vi "Periodic Tasks.vi"(8 "error in":errorcluster) -> ()   [LabVIEW 2014]
doc: "This VI runs in parallel to other tasks. It can contain as many user-defined periodic loops as you need. These can carry out PID or other sorts of timed response."
uses:
  <vilib>/Rock Robotics/WPI/Joystick/WPI_JoystickGetSetRefNum.vi
  <vilib>/Rock Robotics/WPI/RobotDrive/WPI_RobotDriveGetSetRefNum.vi
  Global Variables.vi
  <vilib>/addons/control/pid/NI_PID_pid.lvlib
  <vilib>/addons/control/pid/pid.llb/PID (DBL).vi
panel:
  in  "constant":dbl
  out "encoder counts per iteration 2":dbl format="%#_12g"
  in  "motor speed 2":dbl
  in  "total iterations 2":dbl
  out "iterations":dbl
  out "encoder counts per iteration":dbl format="%#_12g"
  in  "motor speed":dbl
  in  "total iterations":dbl
  out "encoder count left":dbl
  out "encoder count right":dbl
  out "left to target difference":dbl
  out "Waveform Graph 2":dbl[](graph)
  in  "reset graph":bool
  out "Waveform Graph":dbl[](graph)
  in  "move to distance":dbl
  in  "right PID gains":T1={"proportional gain (Kc)"=1.0, "integral time (Ti, min)"=0.01, "derivative time (Td, min)"=0.0} {"derivative time (Td, min)" format="%.4f"; "integral time (Ti, min)" format="%.6f"; "proportional gain (Kc)" format="%.5f"}
  in  "left PID gains":T1={"proportional gain (Kc)"=1.0, "integral time (Ti, min)"=0.01, "derivative time (Td, min)"=0.0} {"derivative time (Td, min)" format="%.10f"; "integral time (Ti, min)" format="%.3f"; "proportional gain (Kc)" format="%.5f"}
  in  "right output range":cluster{"output high":dbl, "output low":dbl}={"output high"=100.0, "output low"=-100.0} {"output low" format="%.2f"; "output high" format="%.2f"}
  in  "left output range":cluster{"output high":dbl, "output low":dbl}={"output high"=100.0, "output low"=-100.0} {"output low" format="%.2f"; "output high" format="%.2f"}
  out "Maximum Difference":dbl
  in  "Distance PID":T1={"proportional gain (Kc)"=1.0, "integral time (Ti, min)"=0.01, "derivative time (Td, min)"=0.0} {"derivative time (Td, min)" format="%.3f"; "integral time (Ti, min)" format="%.3f"; "proportional gain (Kc)" format="%.3f"}
  in  "Difference PID":T1={"proportional gain (Kc)"=1.0, "integral time (Ti, min)"=0.01, "derivative time (Td, min)"=0.0} {"derivative time (Td, min)" format="%.3f"; "integral time (Ti, min)" format="%.3f"; "proportional gain (Kc)" format="%.3f"}
  out "Right Encoder Value":dbl
  out "Left Encoder Value":dbl
  in  "PID gains":T1={"proportional gain (Kc)"=1.0, "integral time (Ti, min)"=0.01, "derivative time (Td, min)"=0.0} {"derivative time (Td, min)" format="%.3f"; "integral time (Ti, min)" format="%.3f"; "proportional gain (Kc)" format="%.3f"}
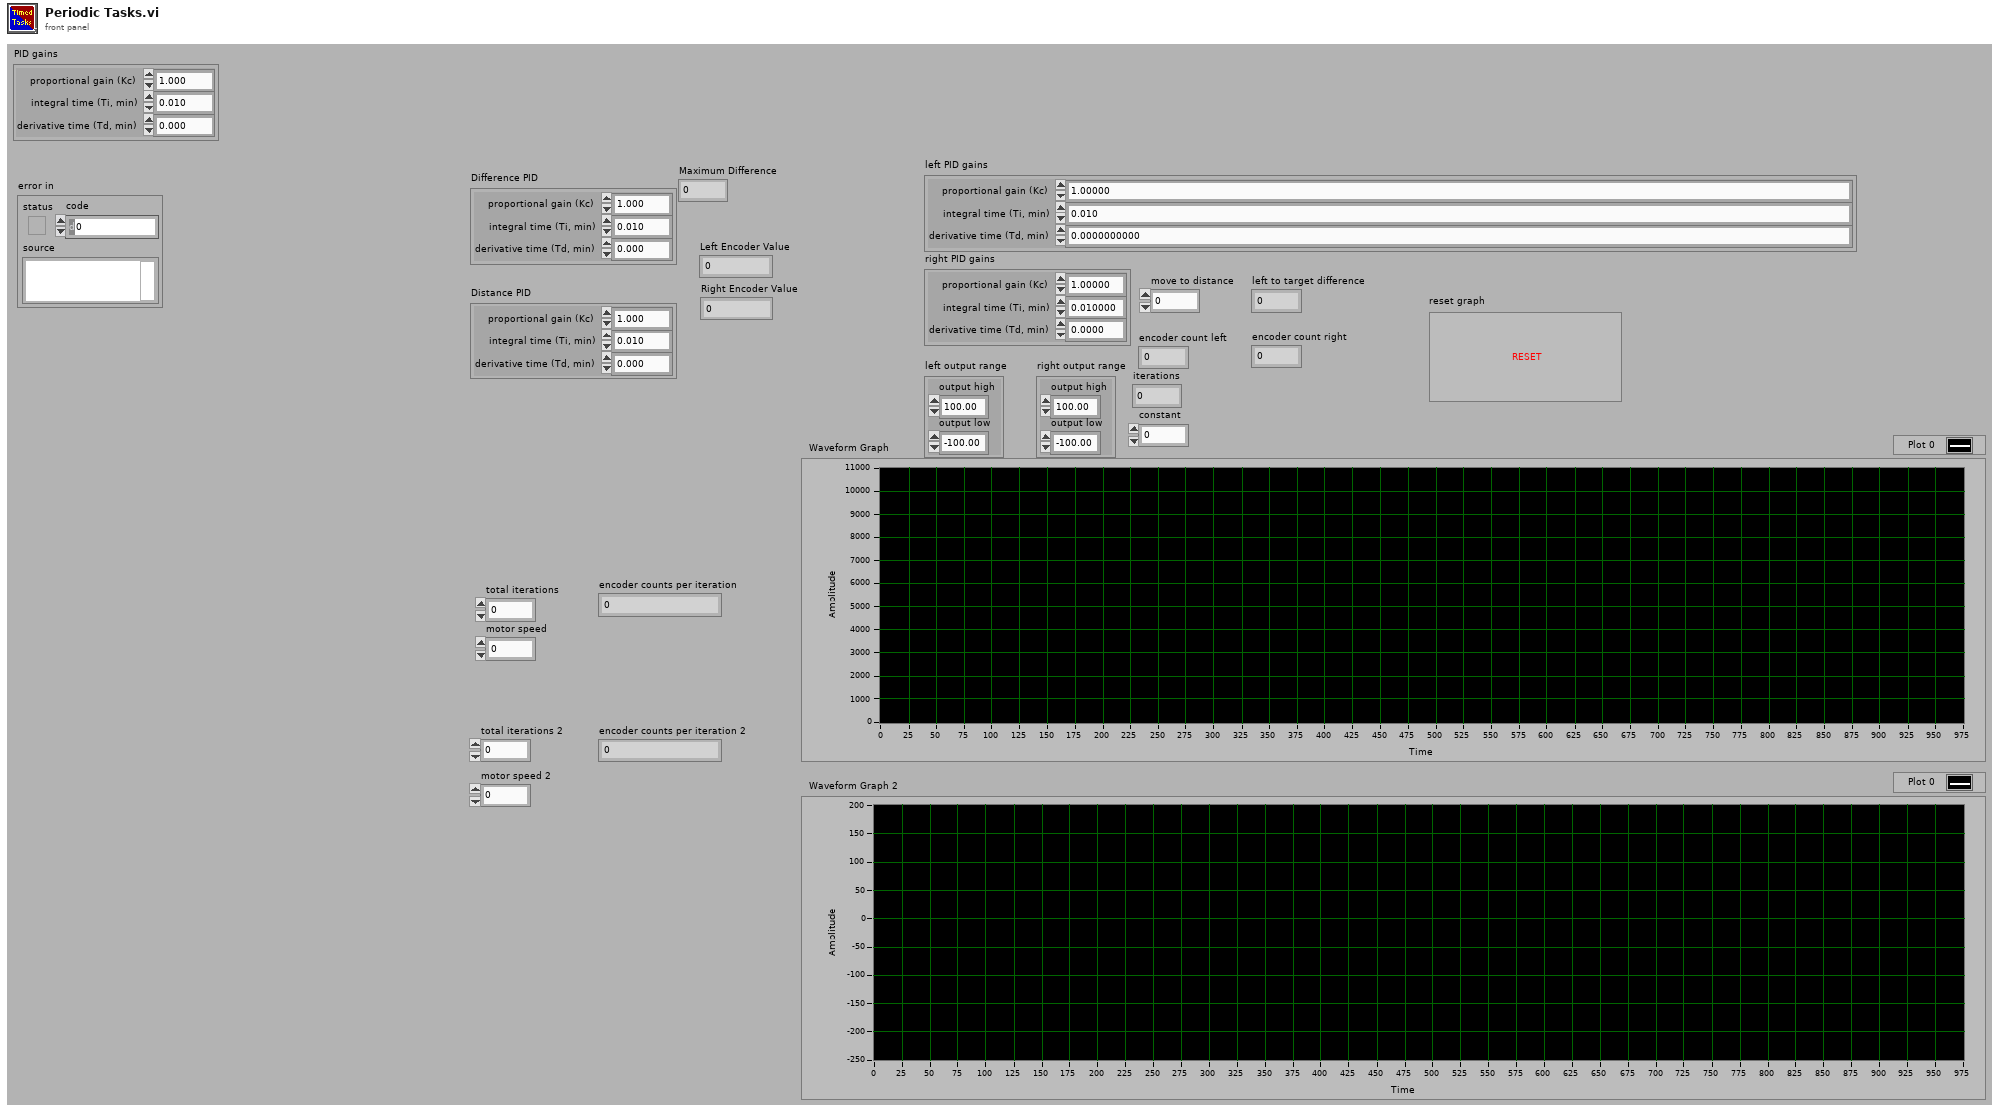
[diagram p1: front panel]
types:
  T1 = cluster{"proportional gain (Kc)":dbl, "integral time (Ti, min)":dbl, "derivative time (Td, min)":dbl}
  T2 = typedef "WPI_JoystickDevRef.ctl" = cluster{"Device":T3}
  T3 = typedef "WPI_JoystickDeviceEnum.ctl" = enum16{"USB 0", "USB 1", "USB 2", "USB 3", "USB 4", "USB 5"}
  T4 = typedef "WPI_RobotDriveDevRef.ctl" = cluster{"DevStatus":errorcluster, "Motors[]":T5[], "Square Inputs":bool, "Max Output":dbl}
  T5 = typedef "WPI_MotorControlDeviceRef.ctl" = cluster{"DeviceStatus":errorcluster, "Type":T6, "PWM":cluster{"Controller":T7, "PWM Channel":T8, "DeadBand":T9}, "CAN":cluster{"Device Number":u8, "Control Mode":T10, "Semaphore":T11, "Max Vout":dbl, "TalonSRX Control Mode":T12}, "Invert":bool, "TransformRef":T13, "InvTransformRef":T13}
  T6 = typedef "WPI_MotorControlType.ctl" = enum16{"PWM", "CAN", "CANTalonSRX"}
  T7 = typedef "FPGA_TypedefDigitalModule.ctl" = enum16{"Controller 1"}
  T8 = typedef "FPGA_DIOPWMChannel.ctl" = enum8{"PWM 0", "PWM 1", "PWM 2", "PWM 3", "PWM 4", "PWM 5", "PWM 6", "PWM 7", "PWM 8", "PWM 9", "PWM MXP 0", "PWM MXP 1", "PWM MXP 2", "PWM MXP 3", "PWM MXP 4", "PWM MXP 5", "PWM MXP 6", "PWM MXP 7", "PWM MXP 8", "PWM MXP 9", "Invalid"}
  T9 = typedef "WPI_PWMDeadband.ctl" = cluster{"Name":string, "maxPositivePwm":i32, "minPositivePwm":i32, "centerPwm":i32, "maxNegativePwm":i32, "minNegativePwm":i32, "angularRange":u16}
  T10 = typedef "WPI_CANJaguar_ControlMode.ctl" = enum8{"Percent VBus", "Current", "Speed", "Position", "Voltage"}
  T11 = typedef "Semaphore RefNum" = refnum<k1>
  T12 = typedef "WPI_CANTalonSRX_APIControlMode.ctl" = enum8{"Percent VBus", "Speed", "Position", "Slave", "Unchanged / Invalid"}
  T13 = typedef "WPI_PWMTransform_ConPane.ctl" = refnum<vi>
  T14 = cluster{"JoystickDevRef":T2, "RobotDriveDevRef":T4}
  T15 = typedef "WPI_EncoderDevRef.ctl" = cluster{"DevStatus":errorcluster, "EncoderIndex":T16, "CounterIndex":T17, "DistancePerCount":dbl, "Decoding Type":T18}
  T16 = typedef "FPGA_EncoderIdx.ctl" = enum8{"Enc 0", "Enc 1", "Enc 2", "Enc 3", "Enc 4", "Enc 5", "Enc 6", "Enc 7", "Invalid"}
  T17 = typedef "FPGA_CounterCtrSystemIndex.ctl" = enum8{"Ctr 0", "Ctr 1", "Ctr 2", "Ctr 3", "Ctr 4", "Ctr 5", "Ctr 6", "Ctr 7", "Invalid"}
  T18 = typedef "WPI_EncoderType.ctl" = enum16{"1x", "2x", "4x"}
  T19 = enum16{"Stop", "Three Tote", "Two Tote", "One Tote", "Step", "Top", "Home", "Joystick", "Joystick Slave", "D Pad"}
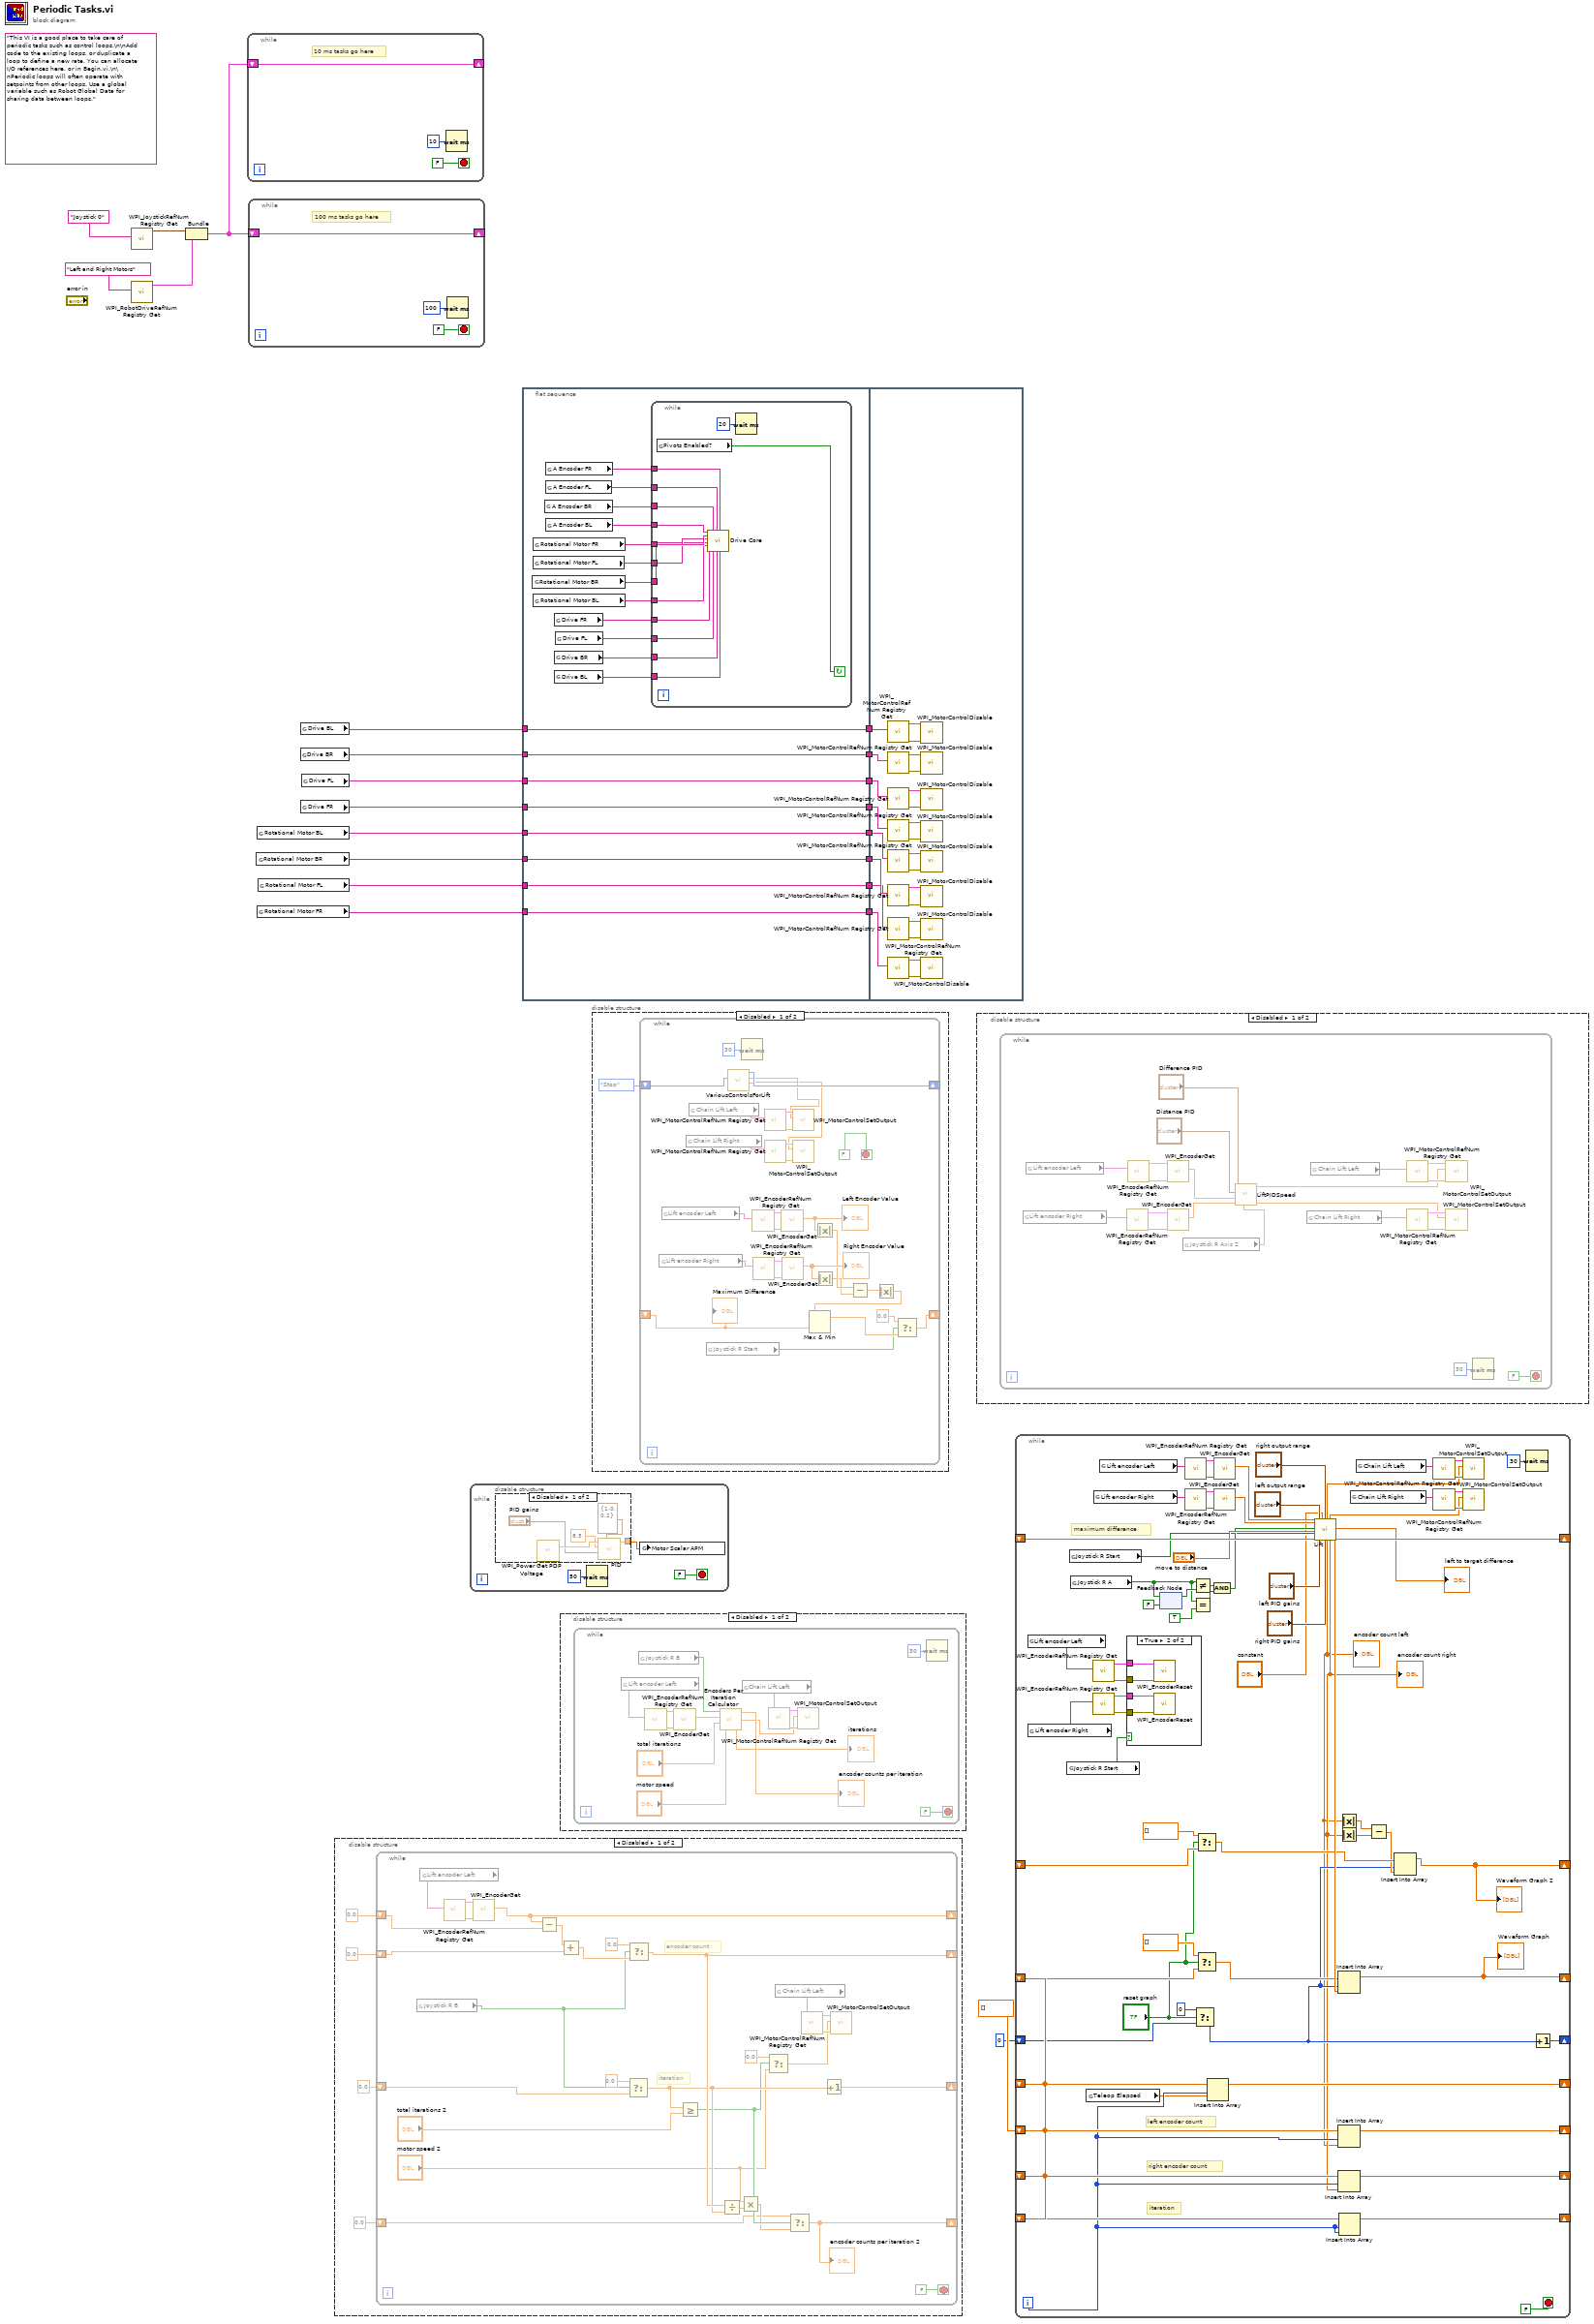
[diagram p0: block diagram]
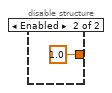
[diagram p7: hidden frame]
diagram:
  w2 = dbl[] []
  (unwired) "This VI is a good place to take care of periodic tasks such as control loops.\n\nAdd code to the existing loops, or duplicate a loop to define a new rate. You can allocate I/O references here, or in Begin.vi.\n\nPeriodic loops will often operate with setpoints from other loops. Use a global variable such as Robot Global Data for sharing data between loops."
  n1 = call <vilib>:"WPI_JoystickRefNum Registry Get.vi"("refnum name"="Joystick 0") -> ("JoystickDevRef"=w21:T2)  [unwired: 1 in, 9 out]
  n2 = call <vilib>:"WPI_RobotDriveRefNum Registry Get.vi"("refnum name"="Left and Right Motors") -> ("RobotDriveDevRef"=w20:T4)  [unwired: 1 in, 9 out]
  n3 = Bundle("JoystickDevRef"=w21, "RobotDriveDevRef"=w20) -> (w19:T14)  [unwired: 1 out]
  n4 = while {
    shift-right: [w24] -> _
    shift-left: w19 -> [w24]
    stop <- FALSE stop-if-true
    # "10 ms tasks go here"
    n5 = Wait (ms)(milliseconds to wait=u32 10) -> ()  [unwired: 1 out]
  }
  n6 = while {
    shift-right: [w27] -> _
    shift-left: w19 -> [w27]
    stop <- FALSE stop-if-true
    # "100 ms tasks go here"
    n7 = Wait (ms)(milliseconds to wait=u32 100) -> ()  [unwired: 1 out]
  }
  n8 = global read "Global Variables.vi" "Rotational Motor BR"() -> (w7:string)
  n9 = global read "Global Variables.vi" "Rotational Motor BL"() -> (w9:string)
  n10 = global read "Global Variables.vi" "Rotational Motor FR"() -> (w3:string)
  n11 = global read "Global Variables.vi" "Rotational Motor FL"() -> (w5:string)
  n12 = global read "Global Variables.vi" "Drive BR"() -> (w15:string)
  n13 = global read "Global Variables.vi" "Drive BL"() -> (w17:string)
  n14 = global read "Global Variables.vi" "Drive FR"() -> (w11:string)
  n15 = global read "Global Variables.vi" "Drive FL"() -> (w13:string)
  n16 = disable-structure shown="Disabled" {
    frame Disabled {
      n17 = while {
        shift-right: [w60] -> _
        shift-left: 0.0 -> [w59]
        shift-right: [w45] -> _
        shift-left: 0.0 -> [w46]
        shift-right: [w50] -> _
        shift-left: 0.0 -> [w51]
        shift-right: [w36] -> _
        shift-left: 0.0 -> [w37]
        stop <- FALSE stop-if-true
        # "iteration"
        # "encoder count"
        n18 = global read "Global Variables.vi" "Joystick R B"() -> (w34:bool)
        n19 = global read "Global Variables.vi" "Lift encoder Left"() -> (w55:string)
        n20 = call <vilib>:"WPI_EncoderRefNum Registry Get.vi"("refnum name"=w55) -> ("error out"=w56:errorcluster, "EncoderDevRef"=w57:T15)  [unwired: 9 in]
        n21 = call <vilib>:"WPI_EncoderGet.vi"("error in (no error)"=w56, "EncoderDevRef"=w57) -> ("Distance"=w50:dbl)  [unwired: 4 in, 5 out]
        n22 = Subtract(x=w50, y=w51) -> (x-y=w49:dbl)
        n23 = Add(x=w49, y=w46) -> (x+y=w48:dbl)
        n24 = Select(t=0.0, s=w34, f=w59) -> (s? t:f=w44:dbl)
        n25 = Select(t=0.0, s=w34, f=w48) -> (s? t:f=w45:dbl)
        n26 = Greater Or Equal?(x=w44, y="total iterations 2") -> (x >= y?=w41:bool)
        n27 = Divide(x=w45, y=w44) -> (x/y=w40:dbl)
        n28 = Multiply(x="motor speed 2", y=w40) -> (x*y=w38:dbl)
        n29 = Select(t=0.0, s=w41, f="motor speed 2") -> (s? t:f=w35:dbl)
        n30 = global read "Global Variables.vi" "Chain Lift Left"() -> (w54:string)
        n31 = Select(t=w37, s=w41, f=w38) -> (s? t:f=w36:dbl)
        "encoder counts per iteration 2" <- w36
        n32 = call <vilib>:"WPI_MotorControlRefNum Registry Get.vi"("refnum name"=w54) -> ("error out"=w52:errorcluster, "MotorControlDevRef"=w53:T5)  [unwired: 9 in]
        n33 = Increment(x=w44) -> (x+1=w60:dbl)
        n34 = call <vilib>:"WPI_MotorControlSetOutput.vi"("error in (no error)"=w52, "Output"=w35, "MotorControlDevRef"=w53) -> ()  [unwired: 6 in, 3 out]
      }
    }
    frame Enabled {
    }
  }
  n35 = while {
    stop <- FALSE stop-if-true
    n36 = disable-structure shown="Disabled" {
      disable-tunnel: [w65 1.0 ("Motor Scalar APM")] -> w62
      frame Disabled {
        n37 = call <vilib>:"WPI_Power Get PDP Voltage.vi"() -> ("voltage (V)"=w68:dbl)  [unwired: 14 in, 1 out]
        n38 = call-poly <vilib>:"PID.vi"("output range"=cluster{"output high":dbl, "output low":dbl} {"output high"=1.0, "output low"=0.2}, "PID gains"="PID gains", "process variable"=8.5 ("setpoint"), "setpoint"=w68) -> ("output"=w65:dbl)  [unwired: 6 in, 1 out]
      }
      frame Enabled {
      }
    }
    n39 = Wait (ms)(milliseconds to wait=u32 50) -> ()  [unwired: 1 out]
    n40 = global write "Global Variables.vi" "Motor Scalar APM"(w62) -> ()
  }
  n41 = flat-sequence {
    tunnel: [w78] -> w18
    tunnel: w17 -> [w78]
    tunnel: [w77] -> w16
    tunnel: w15 -> [w77]
    tunnel: [w76] -> w14
    tunnel: w13 -> [w76]
    tunnel: [w75] -> w12
    tunnel: w11 -> [w75]
    tunnel: [w74] -> w10
    tunnel: w9 -> [w74]
    tunnel: [w73] -> w8
    tunnel: w7 -> [w73]
    tunnel: [w72] -> w6
    tunnel: w5 -> [w72]
    tunnel: [w71] -> w4
    tunnel: w3 -> [w71]
    tunnel: w18 -> [w112]
    tunnel: w16 -> [w111]
    tunnel: w14 -> [w110]
    tunnel: w12 -> [w109]
    tunnel: w10 -> [w108]
    tunnel: w8 -> [w107]
    tunnel: w6 -> [w106]
    tunnel: w4 -> [w105]
    frame #0 {
      n42 = global read "Global Variables.vi" "Rotational Motor BR"() -> (w84:string)
      n43 = global read "Global Variables.vi" "Rotational Motor FR"() -> (w86:string)
      n44 = global read "Global Variables.vi" "Rotational Motor FL"() -> (w85:string)
      n45 = global read "Global Variables.vi" "Rotational Motor BL"() -> (w83:string)
      n46 = global read "Global Variables.vi" "A Encoder BR"() -> (w88:string)
      n47 = global read "Global Variables.vi" "A Encoder FR"() -> (w90:string)
      n48 = global read "Global Variables.vi" "A Encoder FL"() -> (w89:string)
      n49 = global read "Global Variables.vi" "A Encoder BL"() -> (w87:string)
      n50 = global read "Global Variables.vi" "Drive FR"() -> (w82:string)
      n51 = global read "Global Variables.vi" "Drive BR"() -> (w80:string)
      n52 = global read "Global Variables.vi" "Drive BL"() -> (w79:string)
      n53 = global read "Global Variables.vi" "Drive FL"() -> (w81:string)
      n54 = while {
        tunnel: w90 -> [w103]
        tunnel: w89 -> [w102]
        tunnel: w88 -> [w101]
        tunnel: w87 -> [w100]
        tunnel: w86 -> [w99]
        tunnel: w85 -> [w98]
        tunnel: w84 -> [w97]
        tunnel: w83 -> [w96]
        tunnel: w82 -> [w95]
        tunnel: w81 -> [w94]
        tunnel: w80 -> [w93]
        tunnel: w79 -> [w92]
        stop <- w104 continue-if-true
        n55 = global read "Global Variables.vi" "Pivots Enabled?"() -> (w104:bool)
        n56 = call "Drive Core.vi"("A Encoder BL"=w100, "Rotational Motor FR"=w99, "Rotational Motor FL"=w98, "Rotational Motor BR"=w97, "Rotational Motor BL"=w96, "Drive Motor FR"=w95, "A Encoder BR"=w101, "Drive Motor FL"=w94, "A Encoder FL"=w102, "Drive Motor BR"=w93, "A Encoder FR"=w103, "Drive Motor BL"=w92) -> ()  [unwired: 8 in]
        n57 = Wait (ms)(milliseconds to wait=u32 20) -> ()  [unwired: 1 out]
      }
    }
    frame #1 {
      n58 = call <vilib>:"WPI_MotorControlRefNum Registry Get.vi"("refnum name"=w112) -> ("error out"=w128:errorcluster, "MotorControlDevRef"=w127:T5)  [unwired: 9 in]
      n59 = call <vilib>:"WPI_MotorControlRefNum Registry Get.vi"("refnum name"=w111) -> ("error out"=w126:errorcluster, "MotorControlDevRef"=w125:T5)  [unwired: 9 in]
      n60 = call <vilib>:"WPI_MotorControlRefNum Registry Get.vi"("refnum name"=w110) -> ("error out"=w124:errorcluster, "MotorControlDevRef"=w123:T5)  [unwired: 9 in]
      n61 = call <vilib>:"WPI_MotorControlRefNum Registry Get.vi"("refnum name"=w109) -> ("error out"=w122:errorcluster, "MotorControlDevRef"=w121:T5)  [unwired: 9 in]
      n62 = call <vilib>:"WPI_MotorControlRefNum Registry Get.vi"("refnum name"=w108) -> ("error out"=w120:errorcluster, "MotorControlDevRef"=w119:T5)  [unwired: 9 in]
      n63 = call <vilib>:"WPI_MotorControlRefNum Registry Get.vi"("refnum name"=w107) -> ("error out"=w118:errorcluster, "MotorControlDevRef"=w117:T5)  [unwired: 9 in]
      n64 = call <vilib>:"WPI_MotorControlRefNum Registry Get.vi"("refnum name"=w106) -> ("error out"=w116:errorcluster, "MotorControlDevRef"=w115:T5)  [unwired: 9 in]
      n65 = call <vilib>:"WPI_MotorControlRefNum Registry Get.vi"("refnum name"=w105) -> ("error out"=w114:errorcluster, "MotorControlDevRef"=w113:T5)  [unwired: 9 in]
      n66 = call <vilib>:"WPI_MotorControlDisable.vi"("error in (no error)"=w128, "MotorControlDevRef"=w127) -> ()  [unwired: 8 in, 2 out]
      n67 = call <vilib>:"WPI_MotorControlDisable.vi"("error in (no error)"=w126, "MotorControlDevRef"=w125) -> ()  [unwired: 8 in, 2 out]
      n68 = call <vilib>:"WPI_MotorControlDisable.vi"("error in (no error)"=w124, "MotorControlDevRef"=w123) -> ()  [unwired: 8 in, 2 out]
      n69 = call <vilib>:"WPI_MotorControlDisable.vi"("error in (no error)"=w122, "MotorControlDevRef"=w121) -> ()  [unwired: 8 in, 2 out]
      n70 = call <vilib>:"WPI_MotorControlDisable.vi"("error in (no error)"=w120, "MotorControlDevRef"=w119) -> ()  [unwired: 8 in, 2 out]
      n71 = call <vilib>:"WPI_MotorControlDisable.vi"("error in (no error)"=w118, "MotorControlDevRef"=w117) -> ()  [unwired: 8 in, 2 out]
      n72 = call <vilib>:"WPI_MotorControlDisable.vi"("error in (no error)"=w116, "MotorControlDevRef"=w115) -> ()  [unwired: 8 in, 2 out]
      n73 = call <vilib>:"WPI_MotorControlDisable.vi"("error in (no error)"=w114, "MotorControlDevRef"=w113) -> ()  [unwired: 8 in, 2 out]
    }
  }
  n74 = disable-structure shown="Disabled" {
    frame Disabled {
      n75 = while {
        stop <- FALSE stop-if-true
        n76 = global read "Global Variables.vi" "Lift encoder Left"() -> (w143:string)
        n77 = global read "Global Variables.vi" "Joystick R B"() -> (w130:bool)
        n78 = call <vilib>:"WPI_EncoderRefNum Registry Get.vi"("refnum name"=w143) -> ("error out"=w142:errorcluster, "EncoderDevRef"=w141:T15)  [unwired: 9 in]
        n79 = call <vilib>:"WPI_EncoderGet.vi"("error in (no error)"=w142, "EncoderDevRef"=w141) -> ("Distance"=w137:dbl)  [unwired: 4 in, 5 out]
        n80 = call "Encoders Per Iteration Calculator.vi"("motor speed"="motor speed", "total iterations"="total iterations", "encoder count"=w137, "go"=w130) -> ("iterations"=→"iterations":dbl, "motor speed out"=w132:dbl, "encoder counts per iteration"=→"encoder counts per iteration":dbl)
        n81 = global read "Global Variables.vi" "Chain Lift Left"() -> (w138:string)
        n82 = call <vilib>:"WPI_MotorControlRefNum Registry Get.vi"("refnum name"=w138) -> ("error out"=w140:errorcluster, "MotorControlDevRef"=w139:T5)  [unwired: 9 in]
        n83 = call <vilib>:"WPI_MotorControlSetOutput.vi"("error in (no error)"=w140, "Output"=w132, "MotorControlDevRef"=w139) -> ()  [unwired: 6 in, 3 out]
        n84 = Wait (ms)(milliseconds to wait=u32 30) -> ()  [unwired: 1 out]
      }
    }
    frame Enabled {
    }
  }
  n85 = disable-structure shown="Disabled" {
    frame Disabled {
      n86 = while {
        shift-right: [w172] -> _
        shift-left: T19."Stop" ("State Out") -> [w162]
        shift-right: [w148] -> _
        shift-left: _ -> [w149]
        stop <- FALSE stop-if-true
        n87 = global read "Global Variables.vi" "Lift encoder Right"() -> (w156:string)
        n88 = global read "Global Variables.vi" "Lift encoder Left"() -> (w161:string)
        n89 = global read "Global Variables.vi" "Chain Lift Right"() -> (w166:string)
        n90 = global read "Global Variables.vi" "Chain Lift Left"() -> (w167:string)
        n91 = global read "Global Variables.vi" "Joystick R Start"() -> (w145:bool)
        n92 = call "VariousControlsForLift.vi"("State"=w162) -> ("Lift Motor Right"=w163:dbl, "Lift Motor Left"=w168:dbl, "State Out"=w172:T19)  [unwired: 8 in]
        n93 = Wait (ms)(milliseconds to wait=u32 30) -> ()  [unwired: 1 out]
        n94 = call <vilib>:"WPI_EncoderRefNum Registry Get.vi"("refnum name"=w161) -> ("error out"=w160:errorcluster, "EncoderDevRef"=w159:T15)  [unwired: 9 in]
        n95 = call <vilib>:"WPI_EncoderRefNum Registry Get.vi"("refnum name"=w156) -> ("error out"=w157:errorcluster, "EncoderDevRef"=w158:T15)  [unwired: 9 in]
        n96 = call <vilib>:"WPI_MotorControlRefNum Registry Get.vi"("refnum name"=w167) -> ("error out"=w171:errorcluster, "MotorControlDevRef"=w170:T5)  [unwired: 9 in]
        n97 = call <vilib>:"WPI_MotorControlRefNum Registry Get.vi"("refnum name"=w166) -> ("error out"=w164:errorcluster, "MotorControlDevRef"=w165:T5)  [unwired: 9 in]
        n98 = call <vilib>:"WPI_EncoderGet.vi"("error in (no error)"=w160, "EncoderDevRef"=w159) -> ("Distance"=w155:dbl)  [unwired: 4 in, 5 out]
        "Left Encoder Value" <- w155
        n99 = call <vilib>:"WPI_EncoderGet.vi"("error in (no error)"=w157, "EncoderDevRef"=w158) -> ("Distance"=w154:dbl)  [unwired: 4 in, 5 out]
        "Right Encoder Value" <- w154
        n100 = call <vilib>:"WPI_MotorControlSetOutput.vi"("error in (no error)"=w171, "Output"=w168, "MotorControlDevRef"=w170) -> ()  [unwired: 6 in, 3 out]
        n101 = call <vilib>:"WPI_MotorControlSetOutput.vi"("error in (no error)"=w164, "Output"=w163, "MotorControlDevRef"=w165) -> ()  [unwired: 6 in, 3 out]
        n102 = Absolute Value(x=w155) -> (abs(x)=w153:dbl)
        n103 = Absolute Value(x=w154) -> (abs(x)=w152:dbl)
        n104 = Subtract(x=w153, y=w152) -> (x-y=w151:dbl)
        n105 = Absolute Value(x=w151) -> (abs(x)=w150:dbl)
        n106 = Max & Min(x=w150, y=w149) -> (max(x,y)=w146:dbl)  [unwired: 1 out]
        n107 = Select(t=0.0 ("f"), s=w145, f=w146) -> (s? t:f=w148:dbl)
        "Maximum Difference" <- w149
      }
    }
    frame Enabled {
    }
  }
  n108 = disable-structure shown="Disabled" {
    frame Disabled {
      n109 = while {
        stop <- FALSE stop-if-true
        n110 = global read "Global Variables.vi" "Lift encoder Right"() -> (w185:string)
        n111 = global read "Global Variables.vi" "Lift encoder Left"() -> (w188:string)
        n112 = call <vilib>:"WPI_EncoderRefNum Registry Get.vi"("refnum name"=w185) -> ("error out"=w183:errorcluster, "EncoderDevRef"=w184:T15)  [unwired: 9 in]
        n113 = call <vilib>:"WPI_EncoderRefNum Registry Get.vi"("refnum name"=w188) -> ("error out"=w190:errorcluster, "EncoderDevRef"=w189:T15)  [unwired: 9 in]
        n114 = call <vilib>:"WPI_EncoderGet.vi"("error in (no error)"=w183, "EncoderDevRef"=w184) -> ("Distance"=w179:dbl)  [unwired: 4 in, 5 out]
        n115 = call <vilib>:"WPI_EncoderGet.vi"("error in (no error)"=w190, "EncoderDevRef"=w189) -> ("Distance"=w180:dbl)  [unwired: 4 in, 5 out]
        n116 = global read "Global Variables.vi" "Joystick R Axis 2"() -> (w175:dbl)
        n117 = call "LiftPIDSpeed.vi"("joystick"=w175, "right encoder"=w179, "left encoder"=w180, "Distance PID"="Distance PID", "Difference PID"="Difference PID") -> ("Right Motor"=w174:dbl, "Left Motor"=w178:dbl)  [unwired: 5 in]
        n118 = global read "Global Variables.vi" "Chain Lift Right"() -> (w181:string)
        n119 = global read "Global Variables.vi" "Chain Lift Left"() -> (w182:string)
        n120 = call <vilib>:"WPI_MotorControlRefNum Registry Get.vi"("refnum name"=w182) -> ("error out"=w186:errorcluster, "MotorControlDevRef"=w187:T5)  [unwired: 9 in]
        n121 = call <vilib>:"WPI_MotorControlRefNum Registry Get.vi"("refnum name"=w181) -> ("error out"=w192:errorcluster, "MotorControlDevRef"=w191:T5)  [unwired: 9 in]
        n122 = call <vilib>:"WPI_MotorControlSetOutput.vi"("error in (no error)"=w186, "Output"=w178, "MotorControlDevRef"=w187) -> ()  [unwired: 6 in, 3 out]
        n123 = call <vilib>:"WPI_MotorControlSetOutput.vi"("error in (no error)"=w192, "Output"=w174, "MotorControlDevRef"=w191) -> ()  [unwired: 6 in, 3 out]
        n124 = Wait (ms)(milliseconds to wait=u32 30) -> ()  [unwired: 1 out]
      }
    }
    frame Enabled {
    }
  }
  n125 = while {
    shift-right: [w250] -> _
    shift-left: _ -> [w251]
    shift-right: [w237] -> _
    shift-left: w2 -> [w239]
    shift-right: [w236] -> _
    shift-left: w2 -> [w238]
    shift-right: [w226] -> _
    shift-left: w2 -> [w235]
    shift-right: [w220] -> _
    shift-left: w2 -> [w216]
    shift-right: [w223] -> _
    shift-left: w2 -> [w225]
    shift-right: [w219] -> _
    shift-left: 0 -> [w214]
    shift-right: [w207] -> _
    shift-left: _ -> [w212]
    i -> [w224]
    stop <- FALSE stop-if-true
    # "maximum difference"
    # "left encoder count"
    # "right encoder count"
    # "iteration"
    n126 = global read "Global Variables.vi" "Lift encoder Left"() -> (w197:string)
    n127 = global read "Global Variables.vi" "Lift encoder Right"() -> (w196:string)
    n128 = global read "Global Variables.vi" "Joystick R Start"() -> (w198:bool)
    n129 = global read "Global Variables.vi" "Joystick R Start"() -> (w227:bool)
    n130 = global read "Global Variables.vi" "Joystick R A"() -> (w229:bool)
    n131 = global read "Global Variables.vi" "Teleop Elapsed"() -> (w222:dbl)
    n132 = call <vilib>:"WPI_EncoderRefNum Registry Get.vi"("refnum name"=w197) -> ("error out"=w199:errorcluster, "EncoderDevRef"=w200:T15)  [unwired: 9 in]
    n133 = call <vilib>:"WPI_EncoderRefNum Registry Get.vi"("refnum name"=w196) -> ("error out"=w202:errorcluster, "EncoderDevRef"=w201:T15)  [unwired: 9 in]
    n134 = global read "Global Variables.vi" "Lift encoder Right"() -> (w257:string)
    n135 = global read "Global Variables.vi" "Lift encoder Left"() -> (w252:string)
    n136 = case shown="True" w198 {
      tunnel: w202 -> [_ w268]
      tunnel: w201 -> [_ w267]
      tunnel: w199 -> [_ w265]
      tunnel: w200 -> [_ w266]
      frame False {
      }
      frame True {
        n137 = call <vilib>:"WPI_EncoderReset.vi"("error in (no error)"=w265, "EncoderDevRef"=w266) -> ()  [unwired: 8 in, 2 out]
        n138 = call <vilib>:"WPI_EncoderReset.vi"("error in (no error)"=w268, "EncoderDevRef"=w267) -> ()  [unwired: 8 in, 2 out]
      }
    }
    n139 = feedback-in #1(w229) -> ()
    n140 = feedback #1(FALSE ("Joystick R Start")) -> (w234:bool)
    n141 = call <vilib>:"WPI_EncoderRefNum Registry Get.vi"("refnum name"=w252) -> ("error out"=w253:errorcluster, "EncoderDevRef"=w254:T15)  [unwired: 9 in]
    n142 = call <vilib>:"WPI_EncoderRefNum Registry Get.vi"("refnum name"=w257) -> ("error out"=w256:errorcluster, "EncoderDevRef"=w255:T15)  [unwired: 9 in]
    n143 = Not Equal?(x=w229, y=w234) -> (x != y?=w232:bool)
    n144 = Equal?(x=w229, y=TRUE) -> (x = y?=w231:bool)
    n145 = Select(t=0, s="reset graph", f=w214) -> (s? t:f=w208:i32)
    n146 = Select(t=dbl[] [], s="reset graph", f=w212) -> (s? t:f=w210:dbl[])
    n147 = Select(t=dbl[] [], s="reset graph", f=w216) -> (s? t:f=w215:dbl[])
    n148 = Insert Into Array(array=w225, index=w224, new element=w222) -> (w223:dbl[])
    n149 = And(x=w232, y=w231) -> (x .and. y?=w228:bool)
    n150 = call <vilib>:"WPI_EncoderGet.vi"("error in (no error)"=w253, "EncoderDevRef"=w254) -> ("Distance"=w249:dbl)  [unwired: 4 in, 5 out]
    n151 = call <vilib>:"WPI_EncoderGet.vi"("error in (no error)"=w256, "EncoderDevRef"=w255) -> ("Distance"=w248:dbl)  [unwired: 4 in, 5 out]
    n152 = call "Lift.vi"("left encoder"=w249, "right encoder"=w248, "move to"=w228, "move to distance"="move to distance", "reset max"=w227, "last max difference"=w251, "left output range"="left output range", "left PID gains"="left PID gains", "constant"="constant", "right output range"="right output range", "right PID gains"="right PID gains") -> ("lift motor left"=w243:dbl, "encoder count left"=w203:dbl, "lift motor right"=w242:dbl, "encoder count right"=w204:dbl, "left to target difference"=w221:dbl, "max difference"=w250:dbl)  [unwired: 11 in]
    "left to target difference" <- w221
    "encoder count right" <- w204
    "encoder count left" <- w203
    n153 = Absolute Value(x=w203) -> (abs(x)=w206:dbl)
    n154 = Absolute Value(x=w204) -> (abs(x)=w205:dbl)
    n155 = Insert Into Array(array=w215, index=w208, new element=w221) -> (w220:dbl[])
    "Waveform Graph" <- w220
    n156 = Insert Into Array(array=w239, index=w224, new element=w203) -> (w237:dbl[])
    n157 = Insert Into Array(array=w238, index=w224, new element=w204) -> (w236:dbl[])
    n158 = Insert Into Array(array=w235, index=w224, new element=w224) -> (w226:dbl[])
    n159 = global read "Global Variables.vi" "Chain Lift Right"() -> (w261:string)
    n160 = global read "Global Variables.vi" "Chain Lift Left"() -> (w260:string)
    n161 = Subtract(x=w206, y=w205) -> (x-y=w209:dbl)
    n162 = Insert Into Array(array=w210, index=w208, new element=w209) -> (w207:dbl[])
    "Waveform Graph 2" <- w207
    n163 = call <vilib>:"WPI_MotorControlRefNum Registry Get.vi"("refnum name"=w260) -> ("error out"=w258:errorcluster, "MotorControlDevRef"=w259:T5)  [unwired: 9 in]
    n164 = call <vilib>:"WPI_MotorControlRefNum Registry Get.vi"("refnum name"=w261) -> ("error out"=w263:errorcluster, "MotorControlDevRef"=w262:T5)  [unwired: 9 in]
    n165 = call <vilib>:"WPI_MotorControlSetOutput.vi"("error in (no error)"=w258, "Output"=w243, "MotorControlDevRef"=w259) -> ()  [unwired: 6 in, 3 out]
    n166 = call <vilib>:"WPI_MotorControlSetOutput.vi"("error in (no error)"=w263, "Output"=w242, "MotorControlDevRef"=w262) -> ()  [unwired: 6 in, 3 out]
    n167 = Wait (ms)(milliseconds to wait=u32 30) -> ()  [unwired: 1 out]
    n168 = Increment(x=w208) -> (x+1=w219:i32)
  }
